vi "toTestEvent.vi"(10 "assert-store":T2) -> (2 "Assert Event Data":T1={"name"="", "passed"=FALSE, "call-chain"=[], "test-error"={"status"=FALSE, "code"=0, "source"=""}, "timestamp"=timestamp(0 s since 1904-01-01), "assert-id"="", "test-id"="", "time"=-1.0, "message"="", "properties"=variant, "measurements"=variant, "user-defined"=variant})   [LabVIEW 2020, in "Caraya.lvlib" / "Test Event Storage.lvclass"]
uses:
  Test Event Storage.lvclass
  assert store -- cluster.ctl
  Test Manager Message Assertion/TestManagerMsg.Assertion.lvclass
  C:/projects/caraya/src/classes/Test Manager Message/TestManagerMsg.lvclass
  Test Manager Message Verbose/TestManagerMsg.Verbose.lvclass
  Test Result/Assert Event Data (Extended).ctl
  Test Manager Message/TestManagerMsg.lvclass/TestManagerMsg.ctl
  Test Manager Message Verbose/TestManagerMsg.Verbose.lvclass/TestManagerMsg.Verbose.ctl
  Test Manager Message/TestManagerMsg.lvclass
  Test Result/Test Result.lvclass
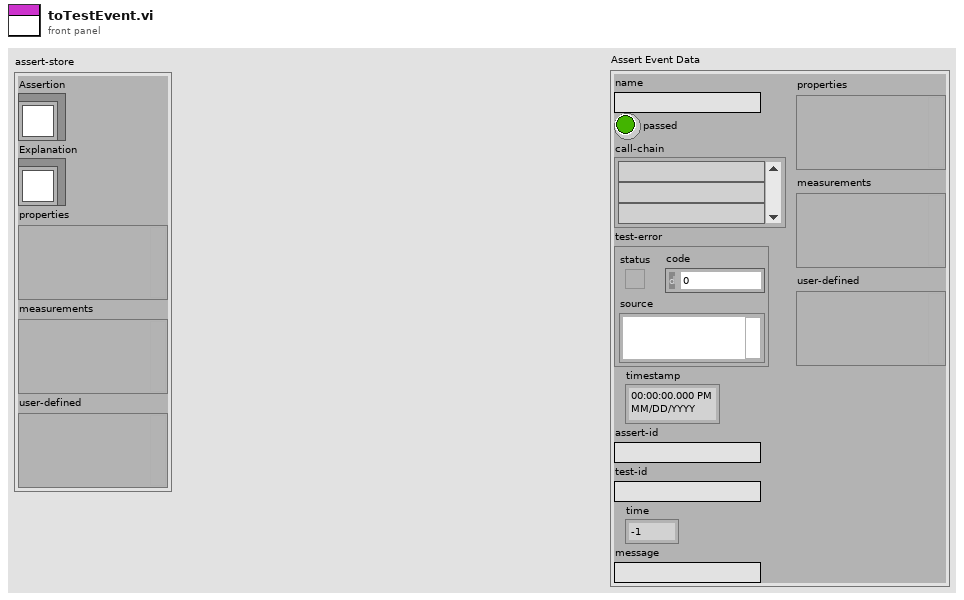
[diagram p1: front panel]
types:
  T1 = typedef "Caraya.lvlib/Test Result.lvclass/Assert Event Data (Extended).ctl" = cluster{"name":string, "passed":bool, "call-chain":string[], "test-error":errorcluster, "timestamp":timestamp, "assert-id":string, "test-id":string, "time":dbl, "message":string, "properties":variant, "measurements":variant, "user-defined":variant}
  T2 = typedef "Caraya.lvlib/Test Event Storage.lvclass/assert store -- cluster.ctl" = cluster{"Assertion":refnum<class "TestManagerMsg.Assertion.lvclass">, "Explanation":refnum<class "TestManagerMsg.Verbose.lvclass">, "properties":variant, "measurements":variant, "user-defined":variant}
  T3 = typedef "Caraya.lvlib/TestManagerMsg.Assertion.lvclass/Assert-Data -- cluster.ctl" = cluster{"Label":string, "Asserted":bool, "call-chain":string[], "upstream-error":errorcluster, "timestamp":timestamp, "Execution time (s)":dbl}
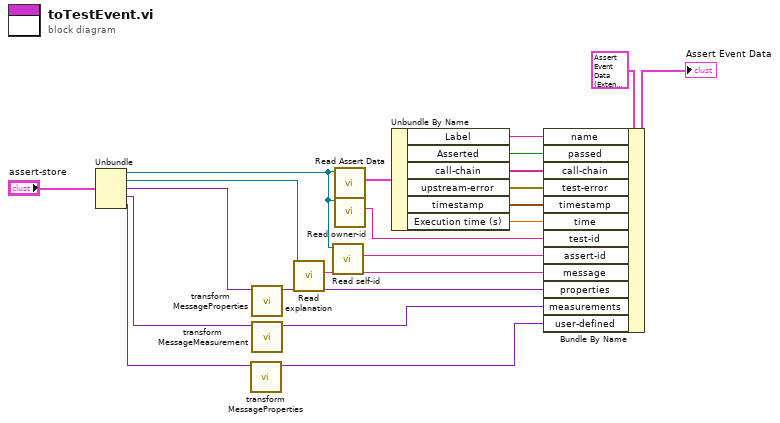
[diagram p0: block diagram]
diagram:
  n1 = Unbundle("assert-store") -> ("Assertion"=w17:refnum<class "TestManagerMsg.Assertion.lvclass">, "Explanation"=w21:refnum<class "TestManagerMsg.Verbose.lvclass">, "properties"=w7:variant, "measurements"=w5:variant, "user-defined"=w2:variant)
  n2 = call "transform MessageProperties.vi"("properties (KVP)"=w2) -> ("properties (Variant Attr)"=w1:variant)  [unwired: 10 in]
  n3 = call "transform MessageProperties.vi"("properties (KVP)"=w7) -> ("properties (Variant Attr)"=w6:variant)  [unwired: 10 in]
  n4 = call "transform MessageMeasurement.vi"("measurements (KVP)"=w5) -> ("measurements (Attributes)"=w4:variant)  [unwired: 10 in]
  n5 = call "Read explanation.vi"("TestManagerMsg.Verbose in"=w21) -> ("explanation"=w20:string)  [unwired: 9 in, 1 out]
  n6 = call "Read self-id.vi"("TestManagerMsg in"=w17) -> ("self-id"=w18:string)  [unwired: 9 in, 1 out]
  n7 = call "Read Assert Data.vi"("Message Assertion"=w17) -> ("Assert Data"=w19:T3)  [unwired: 9 in, 1 out]
  n8 = call "Read owner-id.vi"("TestManagerMsg in"=w17) -> ("owner-id"=w15:string)  [unwired: 9 in, 1 out]
  n9 = Unbundle By Name(w19) -> ("Label"=w10:string, "Asserted"=w11:bool, "call-chain"=w12:string[], "upstream-error"=w13:errorcluster, "timestamp"=w14:timestamp, "Execution time (s)"=w16:dbl)
  n10 = Bundle By Name(cluster=T1 {"name"="", "passed"=FALSE, "call-chain"=[], "test-error"={"status"=FALSE, "code"=0, "source"=""}, "timestamp"=timestamp(0 s since 1904-01-01), "assert-id"="", "test-id"="", "time"=-1.0, "message"="", "properties"=variant, "measurements"=variant, "user-defined"=variant} ("Assert Event Data"), "name"=w10, "passed"=w11, "call-chain"=w12, "test-error"=w13, "timestamp"=w14, "time"=w16, "test-id"=w15, "assert-id"=w18, "message"=w20, "properties"=w6, "measurements"=w4, "user-defined"=w1) -> (→"Assert Event Data":T1)
